vi "Solenoid_Integration.vi"(0 "Number of Samples":dbl, 1 "SampClk.Rate":dbl, 2 "sample mode":i32(ring)=10178 items=["Finite Samples"=10178, "Continuous Samples"=10123, "Hardware Timed Single Point"=12522], 3 "Cluster":T1, 5 "Cluster 2":cluster{dbl, dbl}, 6 "stop":bool, 7 "source":tag, 8 "minimum value":dbl=-10.0 format="%0.2f", 9 "rate":dbl=1000.0 format="%0.2f", 10 "maximum value":dbl=10.0 format="%0.2f") -> (4 "signal out":waveform(dbl)(graph))   [LabVIEW 2021]
uses:
  <vilib>/Utility/error.llb/DialogType.ctl
  <vilib>/DAQmx/write.llb/DAQmx Write (Analog Wfm 1Chan NSamp).vi
  <vilib>/DAQmx/create/channels.llb/DAQmx Create Channel (AO-Voltage-Basic).vi
  <vilib>/DAQmx/configure/timing.llb/DAQmx Timing (Sample Clock).vi
  <vilib>/DAQmx/miscellaneous.llb/DAQmx Fill In Error Info.vi
  <resource>/objmgr/daqmx.rc
  <vilib>/measure/NI_MABase.lvlib
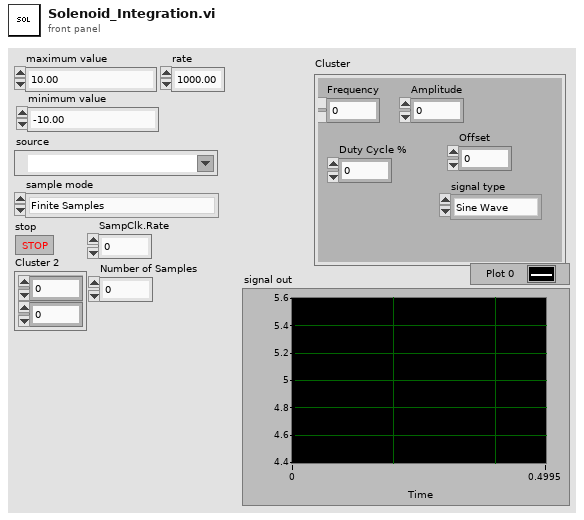
[diagram p1: front panel]
types:
  T1 = cluster{"Frequency":dbl, "Amplitude":dbl, "Duty Cycle %":dbl, "signal type":enum16{"Sine Wave", "Triangle Wave", "Square Wave", "Sawtooth Wave"}, "Offset":dbl}
  T2 = typedef "DialogType.ctl" = u16
  T3 = enum16{"Sine Wave", "Triangle Wave", "Square Wave", "Sawtooth Wave"}
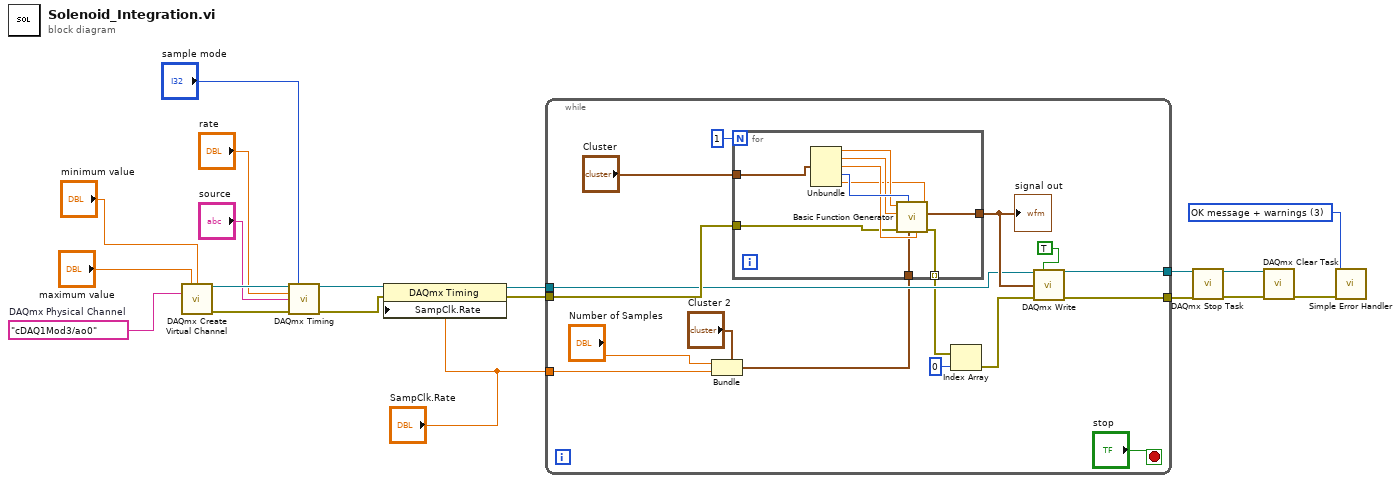
[diagram p0: block diagram]
diagram:
  w1 = T2 3 items=["no dialog", "OK message", "continue or stop message", "OK message + warnings", "continue/stop + warnings"] ("type of dialog (OK msg:1)")
  w19 = tag "cDAQ1Mod3/ao0"  # DAQmx Physical Channel
  n1 = call-poly <vilib>:"DAQmx Create Virtual Channel.vi"("maximum value"="maximum value", "minimum value"="minimum value", "physical channels"=w19) -> ("task out"=w16:refnum<k21>, "error out"=w15:errorcluster)  [unwired: 11 in]
  n2 = call-poly <vilib>:"DAQmx Timing.vi"("task/channels in"=w16, "sample mode"="sample mode", "rate"="rate", "source"="source", "error in"=w15) -> ("task out"=w11:refnum<k21>, "error out"=w10:errorcluster)  [unwired: 9 in]
  n3 = property class="DAQmx Timing"(reference=w11, error in=w10, "SampClk.Rate"="SampClk.Rate") -> (reference out=w8:refnum<k21>, error out=w9:errorcluster)
  n4 = while {
    tunnel: w9 -> [w34]
    tunnel: w8 -> [w32]
    tunnel: "SampClk.Rate" -> [w28]
    tunnel: [w22] -> w6
    tunnel: [w21] -> w5
    stop <- "stop" stop-if-true
    n5 = Bundle(cluster="Cluster 2", "Number of Samples", w28) -> (w27:cluster{dbl, dbl})
    n6 = for {
      N: 1 -> [_]
      tunnel: "Cluster" -> [w45]
      tunnel: [w40] -> w33
      tunnel: w34 -> [w39]
      tunnel: [w38] -> w25 mode=indexing
      tunnel: w27 -> [w37]
      n7 = Unbundle(w45) -> ("Frequency"=w43:dbl, "Amplitude"=w42:dbl, "Duty Cycle %"=w41:dbl, "signal type"=w44:T3, "Offset"=w36:dbl)
      n8 = call <vilib>:"Basic Function Generator.vi"("offset"=w36, "square wave duty cycle (%)"=w41, "sampling info"=w37, "signal type"=w44, "error in (no error)"=w39, "amplitude"=w42, "frequency"=w43) -> ("error out"=w38:errorcluster, "signal out"=w40:waveform(dbl))  [unwired: 2 in, 1 out]
    }
    "signal out" <- w33
    n9 = Index Array(array=w25, index=0) -> (element=w23:errorcluster)
    n10 = call-poly <vilib>:"DAQmx Write.vi"("task/channels in"=w32, "auto start"=TRUE, "data"=w33, "error in"=w23) -> ("task out"=w22:refnum<k21>, "error out"=w21:errorcluster)  [unwired: 9 in, 1 out]
  }
  n11 = call <vilib>:"DAQmx Stop Task.vi"("task/channels in"=w6, "error in"=w5) -> ("task out"=w4:refnum<k21>, "error out"=w3:errorcluster)  [unwired: 12 in]
  n12 = call <vilib>:"DAQmx Clear Task.vi"("task in"=w4, "error in"=w3) -> ("error out"=w2:errorcluster)  [unwired: 13 in]
  n13 = call <vilib>:"Simple Error Handler.vi"("type of dialog (OK msg:1)"=w1, "error in (no error)"=w2) -> ()  [unwired: 3 in, 5 out]
